vi "GetValue.vi"(11 "cluster":T5) -> (3 "output cluster":T1={"Drive"=enum."NI_DAQmx", "TaskType"=enum."AI", "PhysicalChannels"="/Dev1/ai0:3", "SampleRateConfiguration"={"SampleRate"=1000.0, "SamplesPerChannel"=1000, "SamplesPerRead"=200, "SampleMode"=10123, "Clock Source"="OnboardClock"}, "ChannelConfig"="", "Enable"=FALSE} {"SampleRateConfiguration"."SampleMode" items=["Finite Samples"=10178, "Continuous Samples"=10123, "Hardware Timed Single Point"=12522]})   [LabVIEW 2025, in "DAQ_Module.lvlib" / "DAQ_Module.lvclass"]
uses:
  DAQ_Module.lvclass
  DAQ_Module.lvclass/DAQ_Module.ctl
  DAQ_SampleRateConfig.ctl
  DAQ_Task_Type.ctl
  DAQ_HW_Type.ctl
  DAQ_Task_Config.ctl
  eae627af-6bc9-49d6-8f30-d1f4a25a1e11.vi
  b52b4ca5-f496-48f6-8cc4-86826cc6fe67.vi
  ddb27698-2bfe-485e-afc0-30b180fac3f2.vi
  DAQ_Task_UIobject.ctl
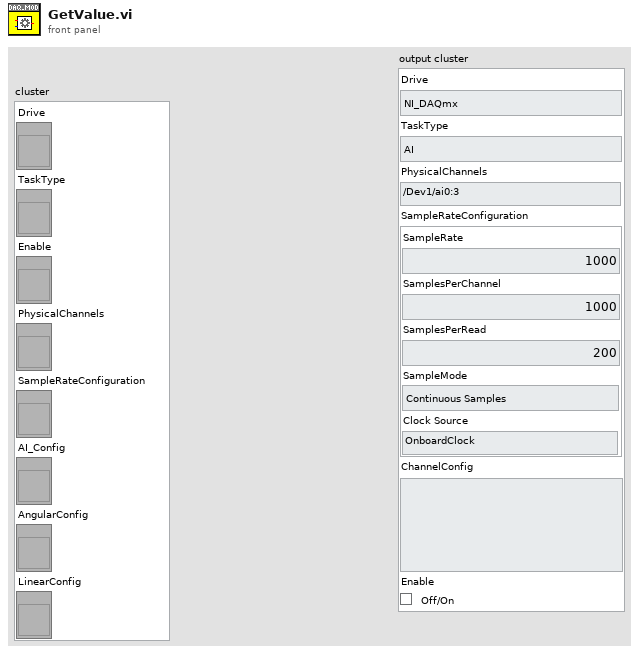
[diagram p1: front panel]
types:
  T1 = typedef "DAQ_Module.lvlib/DAQ_Module.lvclass/DAQ_Task_Config.ctl" = cluster{"Drive":T2, "TaskType":T3, "PhysicalChannels":string, "SampleRateConfiguration":T4, "ChannelConfig":string, "Enable":bool}
  T2 = typedef "DAQ_Module.lvlib/DAQ_Module.lvclass/DAQ_HW_Type.ctl" = enum16{"NI_DAQmx", "Simulated_DAQ"}
  T3 = typedef "DAQ_Module.lvlib/DAQ_Module.lvclass/DAQ_Task_Type.ctl" = enum16{"AI", "Linear", "Angular", "AO"}
  T4 = typedef "DAQ_Module.lvlib/DAQ_Module.lvclass/DAQ_SampleRateConfig.ctl" = cluster{"SampleRate":dbl, "SamplesPerChannel":u32, "SamplesPerRead":i32, "SampleMode":i32, "Clock Source":string}
  T5 = typedef "DAQ_Module.lvlib/DAQ_Module.lvclass/DAQ_Task_UIobject.ctl" = cluster{"Drive":refnum<vi>, "TaskType":refnum<vi>, "Enable":refnum<vi>, "PhysicalChannels":refnum<vi>, "SampleRateConfiguration":refnum<vi>, "AI_Config":refnum<vi>, "AngularConfig":refnum<vi>, "LinearConfig":refnum<vi>}
  T6 = typedef "DAQ_SampleRateConfig.ctl" = cluster{"SampleRate":dbl, "SamplesPerChannel":u32, "SamplesPerRead":i32, "SampleMode":i32, "Clock Source":string}
  T7 = typedef "DAQ_Module.lvlib/DAQ_Module.lvclass/DAQ_AI_Task_Config.ctl" = cluster{"MaxValue":dbl, "MinValue":dbl, "InputTerminalConfiguration":i32}
  T8 = typedef "DAQ_Module.lvlib/DAQ_Module.lvclass/DAQ_Linear_Task_Config.ctl" = cluster{"decoding type":i32, "units":i32, "distance per pulse":dbl, "initial position":dbl, "z index enable":bool, "z index value":dbl, "z index phase":i32, "CI_Encoder_A_InputTerm":string, "CI_Encoder_B_InputTerm":string, "CI_Encoder_Z_InputTerm":string}
  T9 = typedef "DAQ_Module.lvlib/DAQ_Module.lvclass/DAQ_Angular_Task_Config.ctl" = cluster{"decoding type":i32, "units":i32, "pulses per revolution":u32, "initial angle":dbl, "z index enable":bool, "z index value":dbl, "z index phase":i32, "CI_Encoder_A_InputTerm":string, "CI_Encoder_B_InputTerm":string, "CI_Encoder_Z_InputTerm":string}
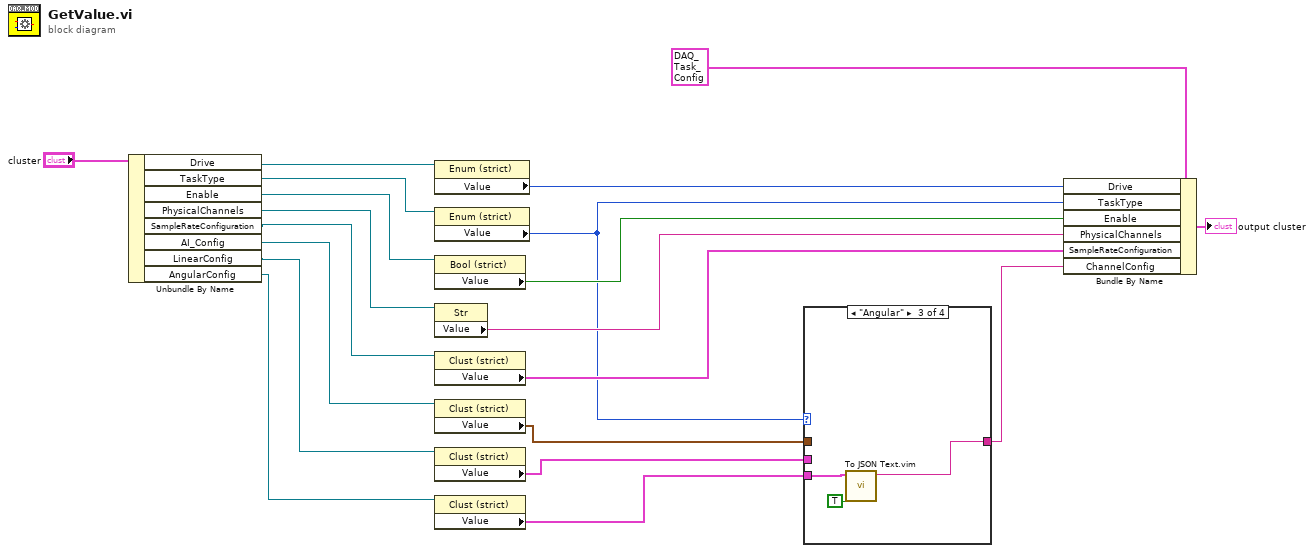
[diagram p0: block diagram]
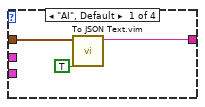
[diagram p2: hidden frame]
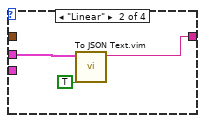
[diagram p3: hidden frame]
diagram:
  n1 = Unbundle By Name("cluster") -> ("Drive"=w19:refnum<vi>, "TaskType"=w18:refnum<vi>, "Enable"=w17:refnum<vi>, "PhysicalChannels"=w16:refnum<vi>, "SampleRateConfiguration"=w15:refnum<vi>, "AI_Config"=w14:refnum<vi>, "LinearConfig"=w7:refnum<vi>, "AngularConfig"=w6:refnum<vi>)
  n2 = property class="Enum (strict)"(reference=w19) -> ("Value"=w12:T2)  [unwired: 1 in, 2 out]
  n3 = property class="Enum (strict)"(reference=w18) -> ("Value"=w8:T3)  [unwired: 1 in, 2 out]
  n4 = property class="Bool (strict)"(reference=w17) -> ("Value"=w11:bool)  [unwired: 1 in, 2 out]
  n5 = property class="Str"(reference=w16) -> ("Value"=w10:string)  [unwired: 1 in, 2 out]
  n6 = property class="Clust (strict)"(reference=w15) -> ("Value"=w9:T6)  [unwired: 1 in, 2 out]
  n7 = property class="Clust (strict)"(reference=w14) -> ("Value"=w5:T7)  [unwired: 1 in, 2 out]
  n8 = property class="Clust (strict)"(reference=w7) -> ("Value"=w4:T8)  [unwired: 1 in, 2 out]
  n9 = property class="Clust (strict)"(reference=w6) -> ("Value"=w3:T9)  [unwired: 1 in, 2 out]
  n10 = case shown="\"Angular\"" w8 {
    tunnel: w5 -> [w22 _ _ _]
    tunnel: [w21 w25 w28 _] -> w2
    tunnel: w4 -> [_ w24 _ _]
    tunnel: w3 -> [_ _ w27 _]
    frame "AI", Default {
      n11 = call "To JSON Text.vim"("Pretty Print?"=TRUE, "Anything"=w22) -> ("<JSON>"=w21:string)  [unwired: 8 in, 1 out]
    }
    frame "Linear" {
      n12 = call "To JSON Text.vim"("Pretty Print?"=TRUE, "Anything"=w24) -> ("<JSON>"=w25:string)  [unwired: 8 in, 1 out]
    }
    frame "Angular" {
      n13 = call "To JSON Text.vim"("Pretty Print?"=TRUE, "Anything"=w27) -> ("<JSON>"=w28:string)  [unwired: 8 in, 1 out]
    }
    frame "AO" {
    }
  }
  n14 = Bundle By Name(cluster=T1 {"Drive"=enum."NI_DAQmx", "TaskType"=enum."AI", "PhysicalChannels"="/Dev1/ai0:3", "SampleRateConfiguration"={"SampleRate"=1000.0, "SamplesPerChannel"=1000, "SamplesPerRead"=200, "SampleMode"=10123, "Clock Source"="OnboardClock"}, "ChannelConfig"="", "Enable"=FALSE} ("value"), "Drive"=w12, "TaskType"=w8, "Enable"=w11, "PhysicalChannels"=w10, "SampleRateConfiguration"=w9, "ChannelConfig"=w2) -> (→"output cluster":T1)
